vi "Smart Helmet_Measurement Project.vi"() -> ()   [LabVIEW 2022 SP3]
uses:
  <vilib>/DAQmx/create/channels.llb/DAQmx Create Channel (AI-Voltage-Basic).vi
  <vilib>/DAQmx/create/channels.llb/DAQmx Create Channel (DO-Digital Output).vi
  <vilib>/DAQmx/write.llb/DAQmx Write (Digital Bool 1Line 1Point).vi
  <vilib>/DAQmx/read.llb/DAQmx Read (Analog 1D DBL NChan 1Samp).vi
panel:
  in  "Notification sender for Impact":tag
  in  "Motor for Alcohol Sensor":tag
  in  "Cooler for Temp Sensor":tag
  in  "stop":bool
  out "Impact":dbl(graph)
  out "Alcohol Level":dbl(graph)
  out "Temperature":dbl(graph)
  in  "physical channels":tag
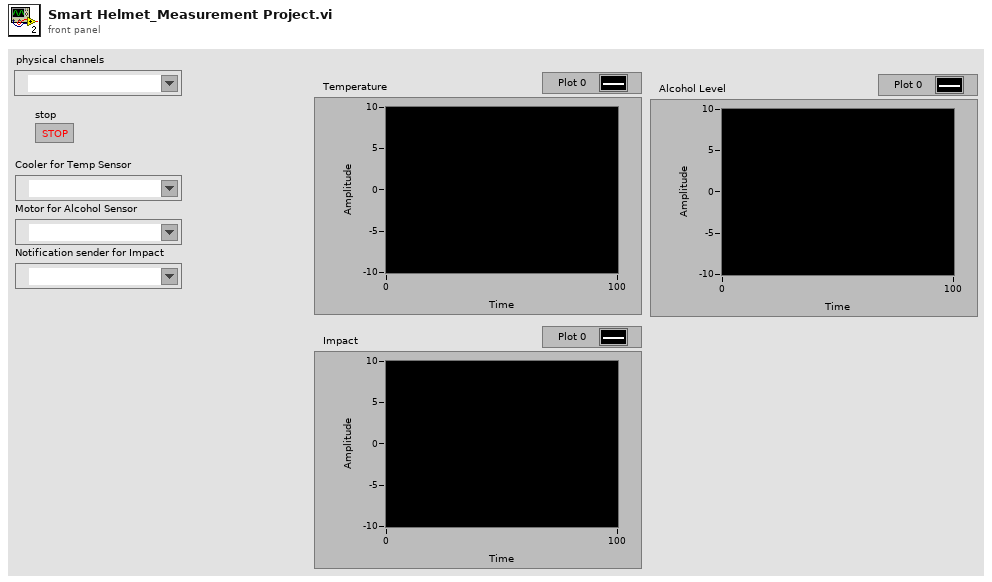
[diagram p1: front panel]
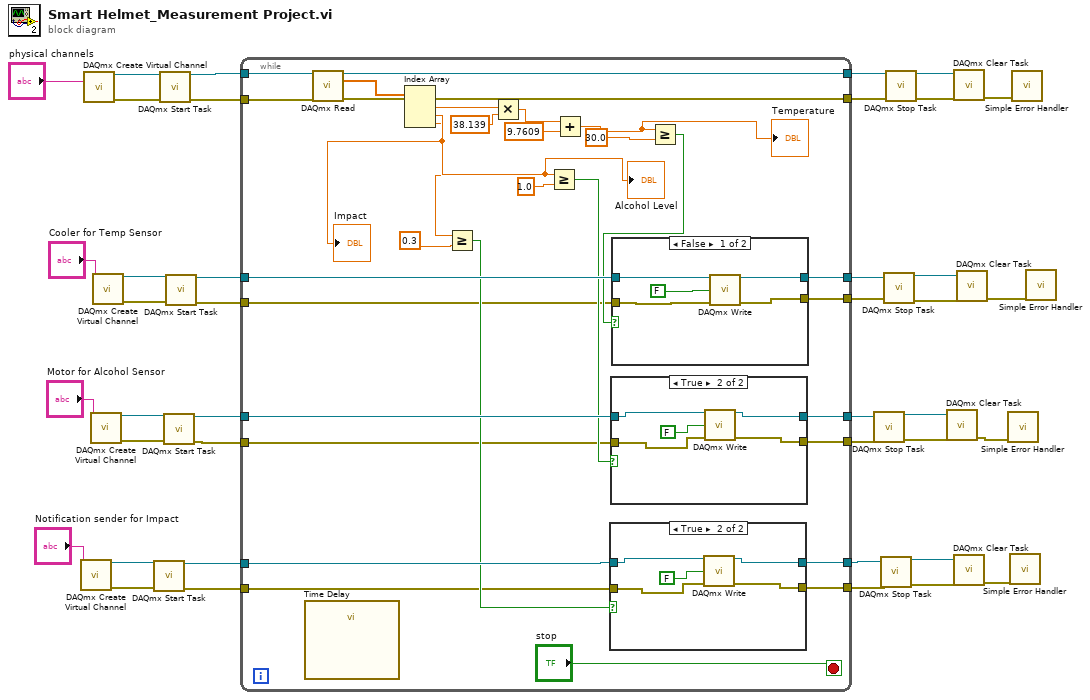
[diagram p0: block diagram]
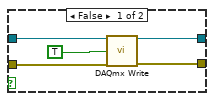
[diagram p2: hidden frame]
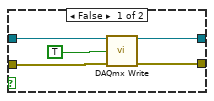
[diagram p3: hidden frame]
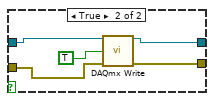
[diagram p4: hidden frame]
diagram:
  n1 = call-poly <vilib>:"DAQmx Create Virtual Channel.vi"("lines"="Notification sender for Impact") -> ("task out"=w25:refnum<k21>, "error out"=w8:errorcluster)  [unwired: 13 in]
  n2 = call-poly <vilib>:"DAQmx Create Virtual Channel.vi"("physical channels"="physical channels") -> ("task out"=w39:refnum<k21>, "error out"=w35:errorcluster)  [unwired: 13 in]
  n3 = call-poly <vilib>:"DAQmx Create Virtual Channel.vi"("lines"="Motor for Alcohol Sensor") -> ("task out"=w27:refnum<k21>, "error out"=w12:errorcluster)  [unwired: 13 in]
  n4 = call-poly <vilib>:"DAQmx Create Virtual Channel.vi"("lines"="Cooler for Temp Sensor") -> ("task out"=w31:refnum<k21>, "error out"=w16:errorcluster)  [unwired: 13 in]
  n5 = call <vilib>:"DAQmx Start Task.vi"("task/channels in"=w25, "error in"=w8) -> ("task out"=w24:refnum<k21>, "error out"=w7:errorcluster)  [unwired: 12 in]
  n6 = call <vilib>:"DAQmx Start Task.vi"("task/channels in"=w39, "error in"=w35) -> ("task out"=w38:refnum<k21>, "error out"=w34:errorcluster)  [unwired: 12 in]
  n7 = call <vilib>:"DAQmx Start Task.vi"("task/channels in"=w27, "error in"=w12) -> ("task out"=w26:refnum<k21>, "error out"=w11:errorcluster)  [unwired: 12 in]
  n8 = call <vilib>:"DAQmx Start Task.vi"("task/channels in"=w31, "error in"=w16) -> ("task out"=w30:refnum<k21>, "error out"=w15:errorcluster)  [unwired: 12 in]
  n9 = while {
    tunnel: w38 -> [w71]
    tunnel: [w62] -> w37
    tunnel: w34 -> [w61]
    tunnel: [w60] -> w33
    tunnel: w30 -> [w56]
    tunnel: [w55] -> w29
    tunnel: w26 -> [w54]
    tunnel: w24 -> [w53]
    tunnel: [w52] -> w22
    tunnel: [w51] -> w20
    tunnel: w15 -> [w46]
    tunnel: [w45] -> w14
    tunnel: w11 -> [w44]
    tunnel: [w43] -> w10
    tunnel: w7 -> [w42]
    tunnel: [w41] -> w6
    stop <- "stop" stop-if-true
    n10 = call "Time Delay"() -> ()  [unwired: 11 in, 1 out]
    n11 = call-poly <vilib>:"DAQmx Read.vi"("task/channels in"=w71, "error in"=w61) -> ("task out"=w62:refnum<k21>, "data"=w70:dbl[], "error out"=w60:errorcluster)  [unwired: 11 in]
    n12 = Index Array(array=w70) -> (element #1=w69:dbl, element #2=w58:dbl, element #3=w57:dbl)  [unwired: 3 in]
    "Alcohol Level" <- w58
    "Impact" <- w57
    n13 = Greater Or Equal?(x=w57, y=0.3) -> (x >= y?=w47:bool)
    n14 = Multiply(x=w69, y=38.139) -> (x*y=w67:dbl)
    n15 = Greater Or Equal?(x=w58, y=1.0) -> (x >= y?=w48:bool)
    n16 = Add(x=w67, y=9.7609) -> (x+y=w59:dbl)
    "Temperature" <- w59
    n17 = case shown="True" w47 {
      tunnel: w53 -> [w76 w81]
      tunnel: [w75 w80] -> w51
      tunnel: w42 -> [w73 w77]
      tunnel: [w72 w78] -> w41
      frame False {
        n18 = call-poly <vilib>:"DAQmx Write.vi"("task/channels in"=w76, "data"=TRUE, "error in"=w73) -> ("task out"=w75:refnum<k21>, "error out"=w72:errorcluster)  [unwired: 10 in, 1 out]
      }
      frame True {
        n19 = call-poly <vilib>:"DAQmx Write.vi"("task/channels in"=w81, "data"=FALSE, "error in"=w77) -> ("task out"=w80:refnum<k21>, "error out"=w78:errorcluster)  [unwired: 10 in, 1 out]
      }
    }
    n20 = case shown="True" w48 {
      tunnel: w54 -> [w86 w91]
      tunnel: [w85 w90] -> w52
      tunnel: w44 -> [w83 w87]
      tunnel: [w82 w88] -> w43
      frame False {
        n21 = call-poly <vilib>:"DAQmx Write.vi"("task/channels in"=w86, "data"=TRUE, "error in"=w83) -> ("task out"=w85:refnum<k21>, "error out"=w82:errorcluster)  [unwired: 10 in, 1 out]
      }
      frame True {
        n22 = call-poly <vilib>:"DAQmx Write.vi"("task/channels in"=w91, "data"=FALSE, "error in"=w87) -> ("task out"=w90:refnum<k21>, "error out"=w88:errorcluster)  [unwired: 10 in, 1 out]
      }
    }
    n23 = Greater Or Equal?(x=w59, y=30.0) -> (x >= y?=w49:bool)
    n24 = case shown="False" w49 {
      tunnel: w56 -> [w96 w101]
      tunnel: [w95 w100] -> w55
      tunnel: w46 -> [w92 w98]
      tunnel: [w93 w97] -> w45
      frame False {
        n25 = call-poly <vilib>:"DAQmx Write.vi"("task/channels in"=w96, "data"=FALSE, "error in"=w92) -> ("task out"=w95:refnum<k21>, "error out"=w93:errorcluster)  [unwired: 10 in, 1 out]
      }
      frame True {
        n26 = call-poly <vilib>:"DAQmx Write.vi"("task/channels in"=w101, "data"=TRUE, "error in"=w98) -> ("task out"=w100:refnum<k21>, "error out"=w97:errorcluster)  [unwired: 10 in, 1 out]
      }
    }
  }
  n27 = call <vilib>:"DAQmx Stop Task.vi"("task/channels in"=w22, "error in"=w10) -> ("task out"=w23:refnum<k21>, "error out"=w9:errorcluster)  [unwired: 12 in]
  n28 = call <vilib>:"DAQmx Stop Task.vi"("task/channels in"=w20, "error in"=w6) -> ("task out"=w21:refnum<k21>, "error out"=w5:errorcluster)  [unwired: 12 in]
  n29 = call <vilib>:"DAQmx Stop Task.vi"("task/channels in"=w29, "error in"=w14) -> ("task out"=w28:refnum<k21>, "error out"=w13:errorcluster)  [unwired: 12 in]
  n30 = call <vilib>:"DAQmx Stop Task.vi"("task/channels in"=w37, "error in"=w33) -> ("task out"=w36:refnum<k21>, "error out"=w32:errorcluster)  [unwired: 12 in]
  n31 = call <vilib>:"DAQmx Clear Task.vi"("task in"=w23, "error in"=w9) -> ("error out"=w2:errorcluster)  [unwired: 13 in]
  n32 = call <vilib>:"DAQmx Clear Task.vi"("task in"=w36, "error in"=w32) -> ("error out"=w4:errorcluster)  [unwired: 13 in]
  n33 = call <vilib>:"DAQmx Clear Task.vi"("task in"=w21, "error in"=w5) -> ("error out"=w1:errorcluster)  [unwired: 13 in]
  n34 = call <vilib>:"DAQmx Clear Task.vi"("task in"=w28, "error in"=w13) -> ("error out"=w3:errorcluster)  [unwired: 13 in]
  n35 = call <vilib>:"Simple Error Handler.vi"("error in (no error)"=w2) -> ()  [unwired: 4 in, 5 out]
  n36 = call <vilib>:"Simple Error Handler.vi"("error in (no error)"=w1) -> ()  [unwired: 4 in, 5 out]
  n37 = call <vilib>:"Simple Error Handler.vi"("error in (no error)"=w4) -> ()  [unwired: 4 in, 5 out]
  n38 = call <vilib>:"Simple Error Handler.vi"("error in (no error)"=w3) -> ()  [unwired: 4 in, 5 out]
